vi "Element Type.vi"(11 "GUI Element in":refnum<class "GUI Element.lvclass">) -> (2 "Element Type":string)   [LabVIEW 2020, in "VolatusGUI.lvlib" / "GUI Element.lvclass"]
uses:
  GUI Element.lvclass
  GUI Element.lvclass/GUI Element.ctl
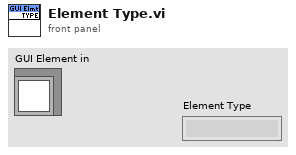
[diagram p1: front panel]
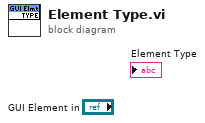
[diagram p0: block diagram]
diagram:
